vi "set Enabled.vi"(10 "Enabled":bool, 11 "Timer in":refnum<class "Timer.lvclass">) -> (3 "Timer out":refnum<class "Timer.lvclass">)   [LabVIEW 2015, in "Timer.lvclass"]
uses:
  Timer.lvclass
  Timer.lvclass/Timer.ctl
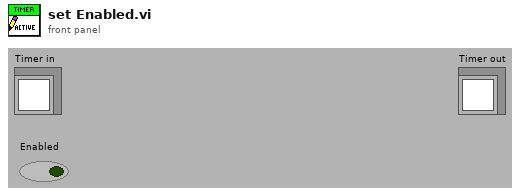
[diagram p1: front panel]
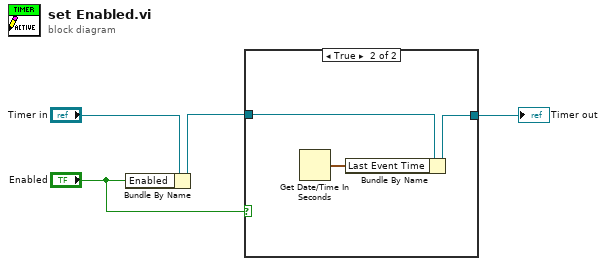
[diagram p0: block diagram]
diagram:
  n1 = Bundle By Name(cluster="Timer in", "Enabled"="Enabled") -> (w3:refnum<class "Timer.lvclass">)
  n2 = case shown="True" "Enabled" {
    tunnel: w3 -> [w5 w8]
    tunnel: [w5 w7] -> w1
    frame False {
    }
    frame True {
      n3 = Get Date/Time In Seconds() -> (seconds since 1Jan1904=w6:timestamp)
      n4 = Bundle By Name(cluster=w8, "Last Event Time"=w6) -> (w7:refnum<class "Timer.lvclass">)
    }
  }
  "Timer out" <- w1
